vi "Test_LogIfError_IncomingError_ErrorLogged.vi"(8 "error in (no error)":errorcluster, 11 "TestCase in":refnum<class "TestLocalLogInstance.lvclass">) -> (0 "error out":errorcluster, 3 "TestCase out":refnum<class "TestLocalLogInstance.lvclass">)   [LabVIEW 2017, in "TestLocalLogInstance.lvclass"]
uses:
  TestLocalLogInstance.lvclass
  Source/Composed Log/Types/Log Level.ctl
  Source/Composed Log/LoggerReference/LoggerReference.lvclass/LoggerReference.ctl
  Source/LVQueue Sink/LVQueue Sink.lvclass/LVQueue Sink.ctl
  4e1641ae-0cdb-4cb3-aa5e-5b59bb93dd62.vi
  Source/Composed Log/LoggerReference/Return Aggregate Queues.vi
  Source/Composed Log/LoggerReference/Add Aggregate Log.vi
  4e1641ae-0cdb-4cb3-aa5e-5b59bb93dd62.vi/1f691d4d-4037-48b6-acf4-7669a2bc2713.vi
  Source/Composed Log/LoggerReference/Send Add Sink.vi
  Source/LVQueue Sink/LVQueue Sink.lvclass
  C:/CS/Internal/LabVIEW/Logger/Source/Composed Log/Log Sink/Log Sink.lvclass
  Source/Composed Log/Application Logger/Launch Worker Loop.vi
  Source/Composed Log/LoggerReference/Initialize Logger Instance.vi
  Source/Composed Log/LoggerReference/LoggerReference.lvclass
  Source/Composed Log/IErrorFormat/IErrorFormat.lvclass
  Source/Composed Log/Log Sink/Log Sink.lvclass
  <vilib>/addons/_JKI Toolkits/VI Tester/TestCase.llb/TestCase.lvclass
  Source/Composed Log/Composed Log.lvlib
  C:/Program Files (x86)/National Instruments/LabVIEW 2017/vi.lib/addons/_JKI Toolkits/VI Tester/TestCase.llb/TestCase.lvclass
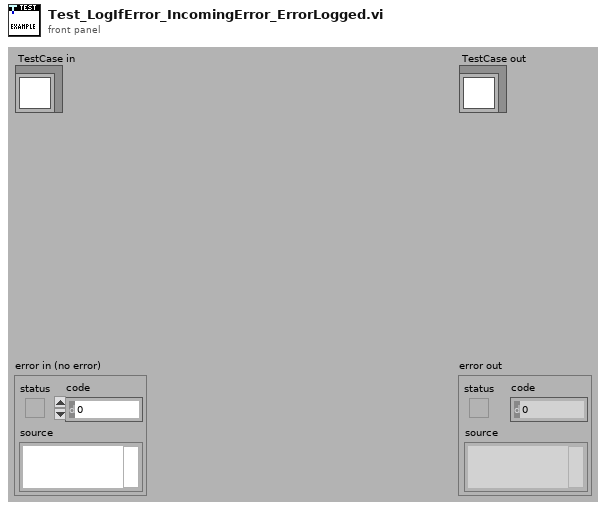
[diagram p1: front panel]
types:
  T1 = typedef "Composed Log.lvlib/Log Level.ctl" = enum16{"Debug", "Info", "Warning", "Error", "Critical"}
  T2 = typedef "Composed Log.lvlib/Log Packet.ctl" = cluster{"Data To Log":string, "Source":string, "Event Level":T1, "Event Time":timestamp}
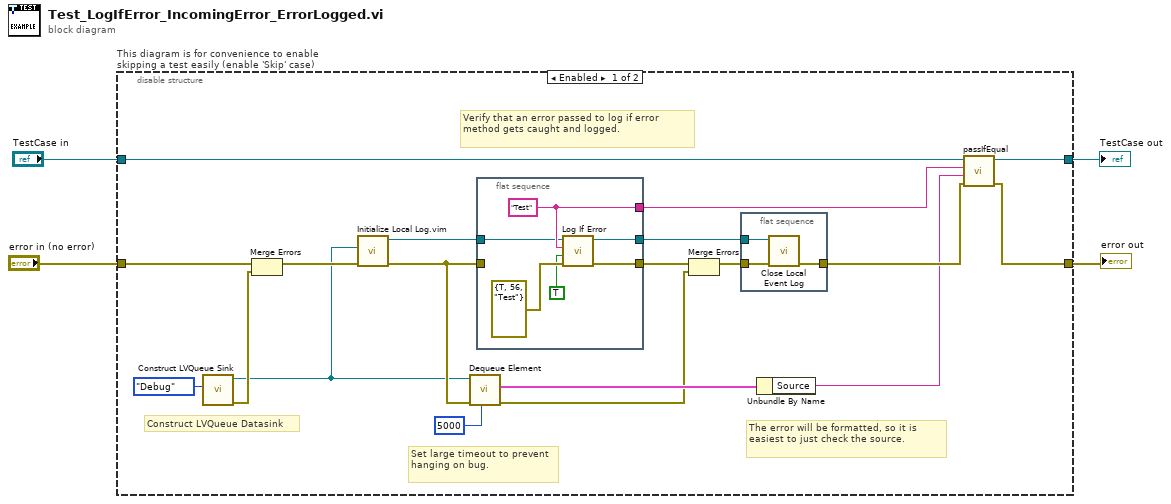
[diagram p0: block diagram]
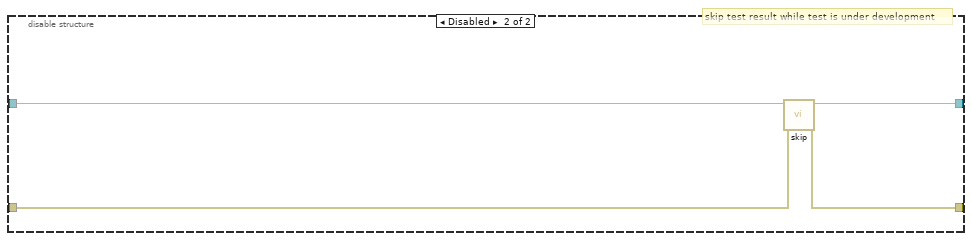
[diagram p2: hidden frame]
diagram:
  n1 = disable-structure "This diagram is for convenience to enable skipping a test easily (enable 'Skip' case)" shown="Enabled" {
    disable-tunnel: "TestCase in" -> [w13 w36]
    disable-tunnel: [w12 w34] -> w1
    disable-tunnel: [w14 w35] -> w3
    disable-tunnel: "error in (no error)" -> [w23 w33]
    frame Enabled {
      # "The error will be formatted, so it is easiest to just check the source."
      # "Construct LVQueue Datasink"
      # "Set large timeout to prevent hanging on bug."
      # "Verify that an error passed to log if error method gets caught and logged."
      n2 = call "Construct LVQueue Sink.vi"("LogLevel"=Log_Level."Debug") -> ("error out"=w19:errorcluster, "LVQueue Sink out"=w7:refnum<class "LVQueue Sink.lvclass">)  [unwired: 9 in]
      n3 = Merge Errors(w23, w19) -> (w9:errorcluster)
      n4 = call "Initialize Local Log.vim"("error in (no error)"=w9, "Startup Sink(s)"=w7) -> ("error out"=w8:errorcluster, "Log Instance Reference"=w6:refnum<class "LoggerReference.lvclass">)  [unwired: 7 in, 1 out]
      n5 = call "Dequeue Element.vi"("timeout in ms (-1)"=5000, "error in (no error)"=w8, "LVQueue Sink in"=w7) -> ("error out"=w17:errorcluster, "Log Packet"=w20:T2)  [unwired: 5 in, 2 out]
      n6 = flat-sequence {
        tunnel: w8 -> [_]
        tunnel: [w28] -> w18
        tunnel: [w27] -> w10
        tunnel: w6 -> [w25]
        tunnel: [w24] -> w5
        frame #0 {
          w27 = "Test" ("SourceID")
          n7 = call "Log If Error.vi"("Error In"=errorcluster {"status"=TRUE, "code"=56, "source"="Test"}, "Clear After Logging?(F)"=TRUE ("Clear Error?(F)"), "SourceID"=w27, "Log Instance"=w25) -> ("error out"=w28:errorcluster, "Log Instance Out"=w24:refnum<class "LoggerReference.lvclass">)  [unwired: 6 in]
        }
      }
      n8 = Merge Errors(w18, w17) -> (w16:errorcluster)
      n9 = flat-sequence {
        tunnel: [w30] -> w15
        tunnel: w16 -> [w32]
        tunnel: w5 -> [w31]
        frame #0 {
          n10 = call "Close Local Event Log.vi"("error in (no error)"=w32, "Log Instance"=w31) -> ("error out"=w30:errorcluster)  [unwired: 9 in]
        }
      }
      n11 = Unbundle By Name(w20) -> ("Source"=w11:string)
      n12 = call-dynamic "passIfEqual.vi"("error in (no error)"=w15, "y"=w11, "x"=w10, "TestCase in"=w13) -> ("error out"=w14:errorcluster, "TestCase out"=w12:refnum<class "TestLocalLogInstance.lvclass">)  [unwired: 6 in]
    }
    frame Disabled {
      # "skip test result while test is under development"
      n13 = call <vilib>:"skip.vi"("error in (no error)"=w33, "TestCase in"=w36) -> ("error out"=w35:errorcluster, "TestCase out"=w34:refnum<class "TestLocalLogInstance.lvclass">)  [unwired: 8 in]
    }
  }
  "error out" <- w3
  "TestCase out" <- w1
